vi "Subvi Shutdown ProSCI.vi"(1 "Current State":i32) -> (0 "Shutdown":bool)   [LabVIEW 2012]
uses:
  ProSCI Global.vi
  <vilib>/Utility/config.llb/Write Key (I32).vi
  <vilib>/Utility/config.llb/NI_LVConfig.lvlib
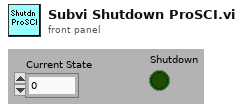
[diagram p1: front panel]
types:
  T1 = typedef "NI_LVConfig.lvlib/Config Data RefNum.ctl" = refnum<k1>
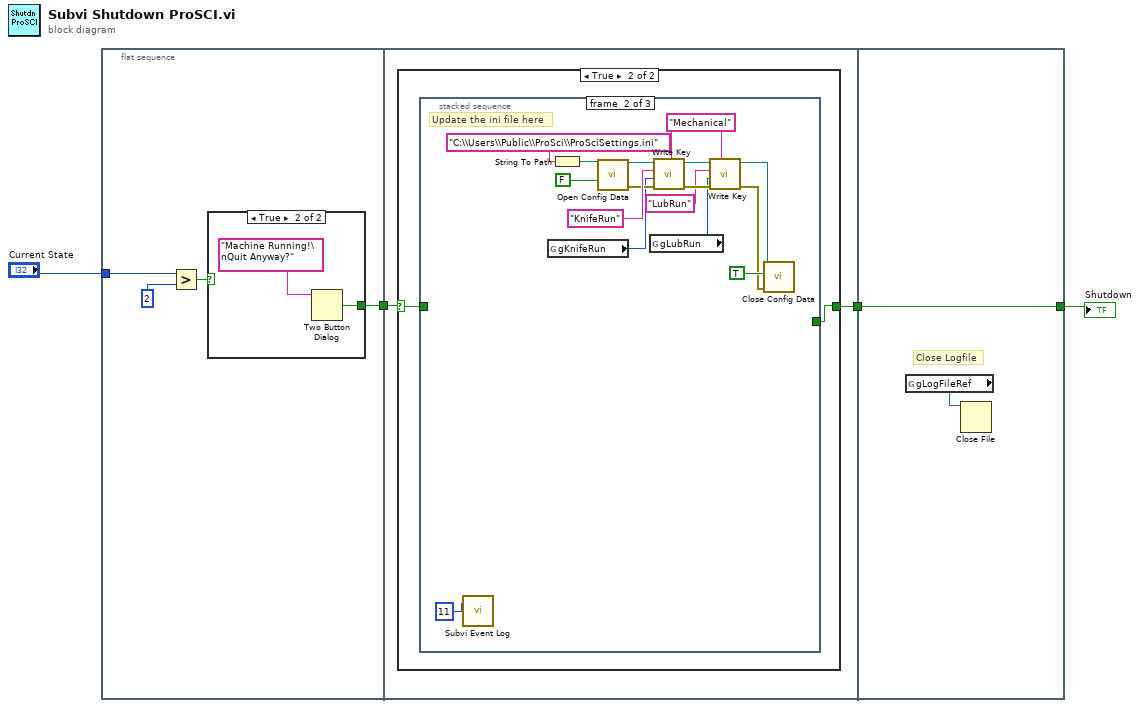
[diagram p0: block diagram]
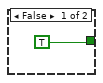
[diagram p2: hidden frame]
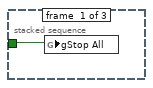
[diagram p4: hidden frame]
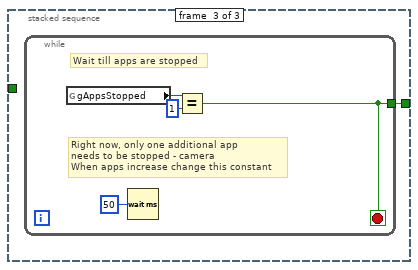
[diagram p5: hidden frame]
diagram:
  n1 = flat-sequence {
    tunnel: [w6] -> w4
    tunnel: "Current State" -> [w5]
    tunnel: w4 -> [w13]
    tunnel: [w12] -> w1
    tunnel: [w40] -> w3
    tunnel: w1 -> [w40]
    frame #0 {
      n2 = Greater?(x=w5, y=2) -> (0:w7:bool)
      n3 = case shown="True" w7 {
        tunnel: [TRUE w10] -> w6
        frame False {
        }
        frame True {
          n4 = Two Button Dialog(message="Machine Running!\nQuit Anyway?") -> (T button?=w10:bool)  [unwired: 2 out]
        }
      }
    }
    frame #1 {
      n5 = case shown="True" w13 {
        selector: w13 -> [w14 w16]
        tunnel: [w14 w15] -> w12
        frame False {
        }
        frame True {
          n6 = stacked-sequence {
            tunnel: w16 -> [w17 _ _]
            tunnel: [_ _ w34] -> w15
            frame #0 {
              n7 = global write "ProSCI Global.vi" "gStop All"(w17) -> ()
            }
            frame #1 {
              w23 = "Mechanical" ("section")
              # "Update the ini file here"
              n8 = call "Subvi Event Log.vi"("EventNum"=u32 11) -> ()  [unwired: 1 in]
              n9 = global read "ProSCI Global.vi" "gKnifeRun"() -> (w21:i32)
              n10 = String To Path(string="C:\\Users\\Public\\ProSci\\ProSciSettings.ini") -> (path=w32:path)
              n11 = call <vilib>:"Open Config Data.vi"("create file if necessary (T)"=FALSE ("create file if necessary? (T)"), "configuration file path"=w32) -> ("error out"=w27:errorcluster, "refnum"=w29:T1)  [unwired: 7 in, 1 out]
              n12 = global read "ProSCI Global.vi" "gLubRun"() -> (w22:i32)
              n13 = call-poly <vilib>:"Write Key.vi"("section"=w23, "error in (no error)"=w27, "value"=w21, "key"="KnifeRun", "refnum"=w29) -> ("error out"=w25:errorcluster, "refnum out"=w26:T1)  [unwired: 5 out]
              n14 = call-poly <vilib>:"Write Key.vi"("section"=w23, "error in (no error)"=w25, "value"=w22, "key"="LubRun", "refnum"=w26) -> ("error out"=w19:errorcluster, "refnum out"=w20:T1)  [unwired: 5 out]
              n15 = call <vilib>:"Close Config Data.vi"("error in (no error)"=w19, "write file if changed (T)"=TRUE ("write configuration file? (T)"), "refnum"=w20) -> ()  [unwired: 9 out]
            }
            frame #2 {
              n16 = while {
                tunnel: [w36] -> w34
                stop <- w36 stop-if-true
                # "Wait till apps are stopped"
                # "Right now, only one additional app\nneeds to be stopped - camera\nWhen apps increase change this constant"
                n17 = global read "ProSCI Global.vi" "gAppsStopped"() -> (w38:u8)
                n18 = Wait (ms)(milliseconds to wait=u32 50) -> ()  [unwired: 1 out]
                n19 = Equal?(x=w38, y=u8 1) -> (x = y?=w36:bool)
              }
            }
          }
        }
      }
    }
    frame #2 {
      # "Close Logfile"
      n20 = global read "ProSCI Global.vi" "gLogFileRef"() -> (w39:refnum<file>)
      n21 = Close File(refnum=w39) -> ()  [unwired: 1 in, 2 out]
    }
  }
  "Shutdown" <- w3
